vi "Get Instance.vi"(8 "error in (no error)":errorcluster, 10 "Create If Not Exist (T)":bool=TRUE, 11 "WebSocket In":refnum<class "Websocket.lvclass">) -> (0 "error out":errorcluster, 1 "NewObjectCreated":bool, 2 "DVRRefOut":refnum<data-value>, 3 "WebSocket Out":refnum<class "Websocket.lvclass">, 5 "ObjectQueueName":string caption="This queue name could be used to destroy\nthe named queue that is used to hold the\nreference in the clean up.")   [LabVIEW 2017, in "Front Panel Publisher.lvlib" / "Websocket.lvclass"]
uses:
  Websocket.lvclass
  Object Attributes.ctl
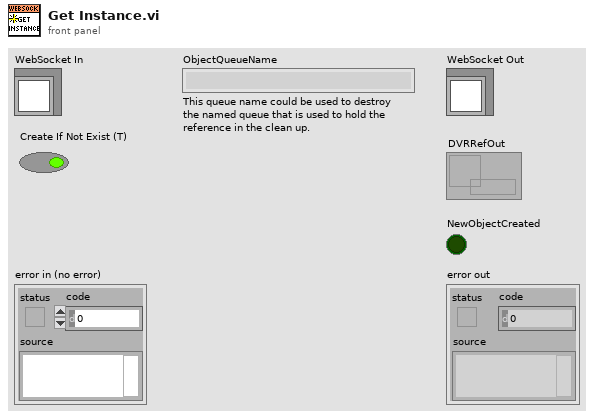
[diagram p1: front panel]
types:
  T1 = enum16{"Create or look up existing", "Look up existing"}
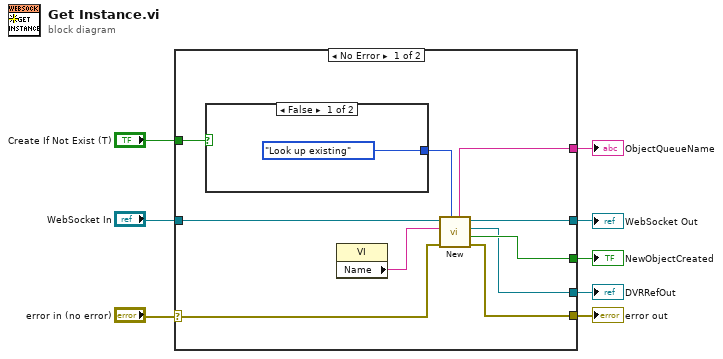
[diagram p0: block diagram]
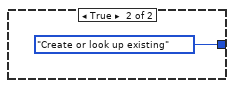
[diagram p2: hidden frame]
diagram:
  n1 = case shown="No Error" "error in (no error)" {
    selector: "error in (no error)" -> [w17 w22]
    tunnel: [w18 w21] -> w8
    tunnel: [w16 w22] -> w6
    tunnel: "WebSocket In" -> [w14 w21]
    tunnel: [w13 _] -> w4
    tunnel: [w12 _] -> w3
    tunnel: [w10 _] -> w2
    tunnel: "Create If Not Exist (T)" -> [w9 _]
    frame No Error {
      n2 = case shown="False" w9 {
        tunnel: [T1."Look up existing" ("CreateMethod(Create or look up existing)") T1."Create or look up existing" ("CreateMethod(Create or look up existing)")] -> w11
        frame False {
        }
        frame True {
        }
      }
      n3 = property class="VI"() -> ("Name"=w15:string)  [unwired: 2 in, 2 out]
      n4 = call "New.vi"("CreateMethod(Create or look up existing)"=w11, "error in (no error)"=w17, "Object name"=w15, "Websocket In"=w14) -> ("error out"=w16:errorcluster, "NewObjectCreated"=w13:bool, "DVRRefOut"=w12:refnum<data-value>, "Websocket Out"=w18:refnum<class "Websocket.lvclass">, "ObjectQueueName"=w10:string)  [unwired: 3 in]
    }
    frame Error {
    }
  }
  "WebSocket Out" <- w8
  "error out" <- w6
  "NewObjectCreated" <- w4
  "DVRRefOut" <- w3
  "ObjectQueueName" <- w2
